vi "file_create_read.vi"(8 "error in (no error)":errorcluster, 11 "config_path":path) -> (0 "error out":errorcluster, 2 "string":string)   [LabVIEW 2015, in "lv-config-json-indexable.lvlib"]
doc: "This file will attempt to open or create a file with read-only permissions, read the entire file and output a string."
uses:
  lv-config-json-indexable.lvlib
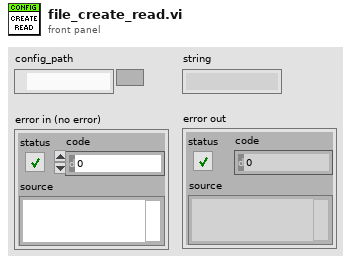
[diagram p1: front panel]
types:
  T1 = enum16{"open", "replace", "create", "open or create", "replace or create", "replace or create with confirmation"}
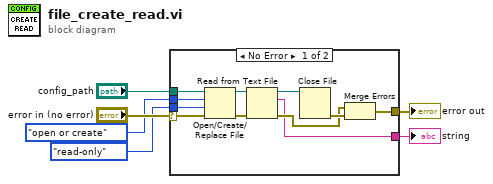
[diagram p0: block diagram]
diagram:
  n1 = case shown="No Error" "error in (no error)" {
    selector: "error in (no error)" -> [w16 w18]
    tunnel: "config_path" -> [w15 _]
    tunnel: [w10 w18] -> w4
    tunnel: [w9 _] -> w3
    tunnel: T1."open or create" ("operation (0:open)") -> [w8 _]
    tunnel: enum16{"read/write", "read-only", "write-only"}."read-only" ("access (0:read/write)") -> [w7 _]
    frame No Error {
      n2 = Open/Create/Replace File(file path (use dialog)=w15, error in=w16, operation (0:open)=w8, access (0:read/write)=w7) -> (refnum out=w12:refnum<file>, error out=w13:errorcluster)  [unwired: 2 in, 1 out]
      n3 = Read from Text File(file (use dialog)=w12, error in=w13) -> (refnum out=w11:refnum<file>, text=w9:string, error out=w14:errorcluster)  [unwired: 2 in, 1 out]
      n4 = Close File(refnum=w11) -> (error out=w17:errorcluster)  [unwired: 1 in, 1 out]
      n5 = Merge Errors(w14, w17) -> (w10:errorcluster)
    }
    frame Error {
    }
  }
  "error out" <- w4
  "string" <- w3
